vi "GetAcqSeqLeCroy.vi"(0 "Digitizer Settings":T5={"Digitizer delay (us) "=0.0, "rf points per line"=2048, "lines per plane"=128, "Samp Rate (Hz)"=100000000.0, "Additional dig delay (us)"=0.0, "Voltage Scale"=0.4, "Pre-Looks"=0, "Offset delay (us)"=0.0, "bits A/D"=8, "Avg Num"=1, "DigTimeOut"=5.0, "Rel Dig Delay"=0.0, "Dig Ch"=0, "LeCroyCluster"={"LeCroy Channels"=[TRUE, FALSE, FALSE, FALSE], "LC read pt offset"=0.0, "Sweep Avg"=FALSE}, "Main Digitizer"=enum."NI Digitizer", "Dig Config"=enum."Single channel", "Digitizer ID Cluster"={"Acqiris/Alazar/SP ID"=[], "NI Instr Handles"=[], "LeCroy VISA"="", "GaGe Handle"={"Handle"=0, "Sample size"=0, "Resolution"=0, "Offset"=0, "Channels"=0, "Boards"=0}, "ATS Ref"="ATS9350", "Acqiris Address"=["PCI::INSTR0"], "ADQRef"=refnum, "adq_cu_ptr"=refnum}, "Trigger Settings"={"Trig Source"=1, "Trig Coupling"=0, "Trig Slope"=0, "Level (mV)"=1500.0}, "Bulk Acq"=FALSE, "Bulk Start Indexes"=[], "Data Ref RF"=refnum, "NI ID/Channel"=[], "Total Dig CH"=1, "Xtra Ann Trig delay (us)"=10.0, "Fix Z Delay?"=FALSE, "One Way Transmission?"=FALSE, "Data Ref Log"=refnum} {"Trigger Settings"."Trig Slope" items=["Positive", "Negative"]; "Trigger Settings"."Level (mV)" format="%.2f"; "Trigger Settings"."Trig Coupling" items=["DC 1 MOhm", "AC 1 MOhm", "DC 50 Ohm", "AC 50 Ohm"]; "Trigger Settings"."Trig Source" items=["Chan 1", "External"]; "Rel Dig Delay" format="%.2f"; "DigTimeOut" format="%.2f"; "Avg Num" min=1; "Offset delay (us)" format="%.2f"; "Additional dig delay (us)" format="%.2f"; "Digitizer delay (us)" format="%.2f"}, 6 "Motion Settings":T1={"No Motion?"=FALSE, "Motion System"=enum."NI 735x", "Motion Bd ID"=1, "Motion Profile"="SMAC1", "# Axis"=1, "Reverse Z axis?"=TRUE, "SMAC Axis"=0, "scan pair"=enum."y-(x) scan", "RT fps"=6.0, "Steps per mm"=[1000, 1000, 1000, 1000], "Motor Parameters"={"velocity ct/s"=[10000.0, 10000.0, 10000.0, 50000.0], "accel ct/s^2"=[50000.0, 50000.0, 50000.0, 200000.0]}, "One Way Scan"=FALSE, "Reverse One Way Scan"=FALSE, "Global Position (mm)"=[], "Plane"=0, "Distance between\nscan lines (um)"=0.0, "Distance between\nscan planes (um)"=0.0, "number of scan planes"=1, "Total steps in line"=0, "Xtra plane\ndistance  (um)"=100, "Xtra planes "=1, "Add Axis"=FALSE, "overshoot cts"=200, "BKPT Shift"=0, "Scan Start Time (ms)"=0, "ESP VISA"="GPIB::1::INSTR", "3rd Axis"=1, "GL Ref Out"=refnum, "Galil Address"=""} {"3rd Axis" items=["x", "y", "z", "w"]; "Xtra planes" min=1; "Xtra plane\ndistance  (um)" min=0; "Distance between\nscan planes (um)" format="%.2f"; "Distance between\nscan lines (um)" format="%.2f"; "SMAC Axis" items=["None"=0, "Axis 1"=1, "Axis 2"=2, "Axis 3"=3, "Axis 4"=4, "Axis 5"=5, "Axis 6"=6, "Axis 7"=7, "Axis 8"=8, "Vector Space 1"=17, "Vector Space 2"=18, "Vector Space 3"=19, "Vector Space 4"=20]; "Motion Bd ID" min=1 max=32 step=1}, 7 "errorin":errorcluster, 8 "Numbered File":string, 9 "Pop Up":bool, 11 "Source (0: Channel 1)":u16(ring) items=["Channel 1", "Channel 2", "Channel 3", "Channel 4", "Memory 1", "Memory 2", "Memory 3", "Memory 4", "Function 1", "Function 2", "Function 3", "Function 4", "Function 5", "Function 6", "Function 7", "Function 8", "Other"], 14 "save?":bool=TRUE, 15 "Reverse?":bool) -> (17 "Raw VGain (scale)":dbl, 18 "Voltage Scale":T9, 20 "Data Array":i16[][](array[numeric]), 21 "VGain (dB)":dbl, 25 "Ch1 Hz Offset":dbl[](array[numeric]), 26 "Ch2 Hz Offset":dbl[](array[numeric]), 27 "error out":errorcluster)   [LabVIEW 2022 SP3]
uses:
  -DigitizerRoutines/DigitizerSettings.ctl
  -DigitizerRoutines/Digitizer.ctl
  -DigitizerRoutines/DigConfig.ctl
  -DigitizerRoutines/DigitizerID.ctl
  C:/Windows/System32/ADQAPI_dotNet_helper.dll
  Motion Controllers/NI_controller/-NI_MotionRoutines/MotionParameters.ctl
  Motion Controllers/NI_controller/-NI_MotionRoutines/MotionSys.ctl
  Motion Controllers/-MotionRoutines/ScanAxis.ctl
  Motion Controllers/-MotionRoutines/3rdAxis.ctl
  -DigitizerRoutines/DigitizerGlobals.vi
  Motion Controllers/-MotionRoutines/MotionGlobals.vi
  <vilib>/Utility/file.llb/Write Delimited Spreadsheet (DBL).vi
  <instrlib>/LeCroy Wave Series/LeCroy Wave Series.lvlib
panel:
  out "Run Time":sgl
  in  "Timeout (10000 ms)":u32=10000
  in  "Sparsing (0: Every point)":i16
  # "1-D and 2-D B scan settings"
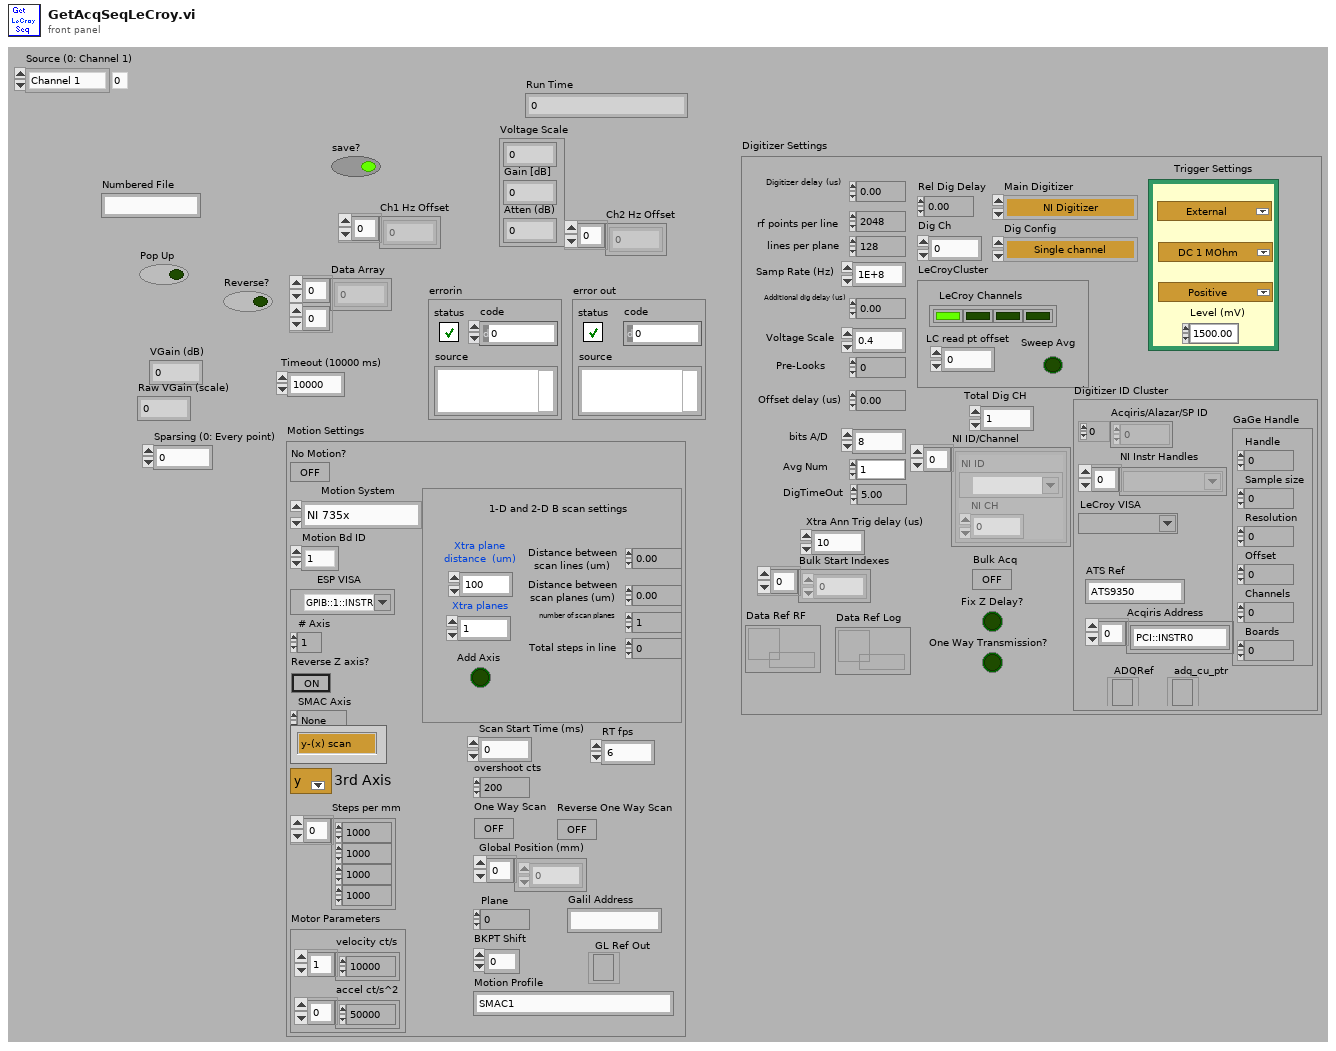
[diagram p1: front panel]
types:
  T1 = typedef "MotionParameters.ctl" = cluster{"No Motion?":bool, "Motion System":T2, "Motion Bd ID":u8, "Motion Profile":string, "# Axis":i8, "Reverse Z axis?":bool, "SMAC Axis":u16, "scan pair":T3, "RT fps":sgl, "Steps per mm":i32[], "Motor Parameters":cluster{"velocity ct/s":dbl[], "accel ct/s^2":dbl[]}, "One Way Scan":bool, "Reverse One Way Scan":bool, "Global Position (mm)":dbl[], "Plane":i32, "Distance between\nscan lines (um)":sgl, "Distance between\nscan planes (um)":sgl, "number of scan planes":i32, "Total steps in line":i32, "Xtra plane\ndistance  (um)":i32, "Xtra planes ":i32, "Add Axis":bool, "overshoot cts":i32, "BKPT Shift":i32, "Scan Start Time (ms)":u32, "ESP VISA":refnum<visa-resource-name>, "3rd Axis":T4, "GL Ref Out":refnum<k7>, "Galil Address":string}
  T2 = typedef "MotionSys.ctl" = enum16{"MM3000", "NI 735x", "Newport ESP", "No Motion Card", "Galil"}
  T3 = typedef "ScanAxis.ctl" = enum16{"y-(x) scan", "x-(y) scan", "z-(x) scan", "z-(y) scan", "y-(z) scan", "x-(z) scan", "w-(x) scan", "w-(y) scan", "w-(z) scan", "x-(w) scan", "y-(w) scan", "z-(w) scan"}
  T4 = typedef "3rdAxis.ctl" = u16
  T5 = typedef "DigitizerSettings.ctl" = cluster{"Digitizer delay (us) ":dbl, "rf points per line":i32, "lines per plane":i32, "Samp Rate (Hz)":dbl, "Additional dig delay (us)":dbl, "Voltage Scale":dbl, "Pre-Looks":i32, "Offset delay (us)":dbl, "bits A/D":i8, "Avg Num":i32, "DigTimeOut":sgl, "Rel Dig Delay":sgl, "Dig Ch":i32, "LeCroyCluster":cluster{"LeCroy Channels":bool[], "LC read pt offset":dbl, "Sweep Avg":bool}, "Main Digitizer":T6, "Dig Config":T7, "Digitizer ID Cluster":T8, "Trigger Settings":cluster{"Trig Source":u16, "Trig Coupling":u16, "Trig Slope":u16, "Level (mV)":dbl}, "Bulk Acq":bool, "Bulk Start Indexes":i32[], "Data Ref RF":refnum<data-value>, "NI ID/Channel":cluster{"NI ID":refnum<k15>, "NI CH":i32}[], "Total Dig CH":i32, "Xtra Ann Trig delay (us)":dbl, "Fix Z Delay?":bool, "One Way Transmission?":bool, "Data Ref Log":refnum<data-value>}
  T6 = typedef "Digitizer.ctl" = enum16{"Acqiris Digitizer", "NI Digitizer", "LeCroy", "GaGe", "AlazarTech", "No Digitizer", "Teledyne"}
  T7 = typedef "DigConfig.ctl" = enum16{"Single channel", "2 Chans w/ 2 Acqiris", "2 Chans w/ 1 Acqiris", "5-CH Pulser New", "5-CH pulser w/ ann array", "5-pass style ann array", "Empty"}
  T8 = typedef "DigitizerID.ctl" = cluster{"Acqiris/Alazar/SP ID":u32[], "NI Instr Handles":refnum<k15>[], "LeCroy VISA":refnum<visa-resource-name>, "GaGe Handle":cluster{"Handle":u32, "Sample size":u32, "Resolution":i32, "Offset":i32, "Channels":u32, "Boards":u32}, "ATS Ref":string, "Acqiris Address":string[], "ADQRef":refnum<k24>, "adq_cu_ptr":refnum<k24>}
  T9 = cluster{sgl, "Gain [dB]  ":sgl, "Atten (dB)":sgl}
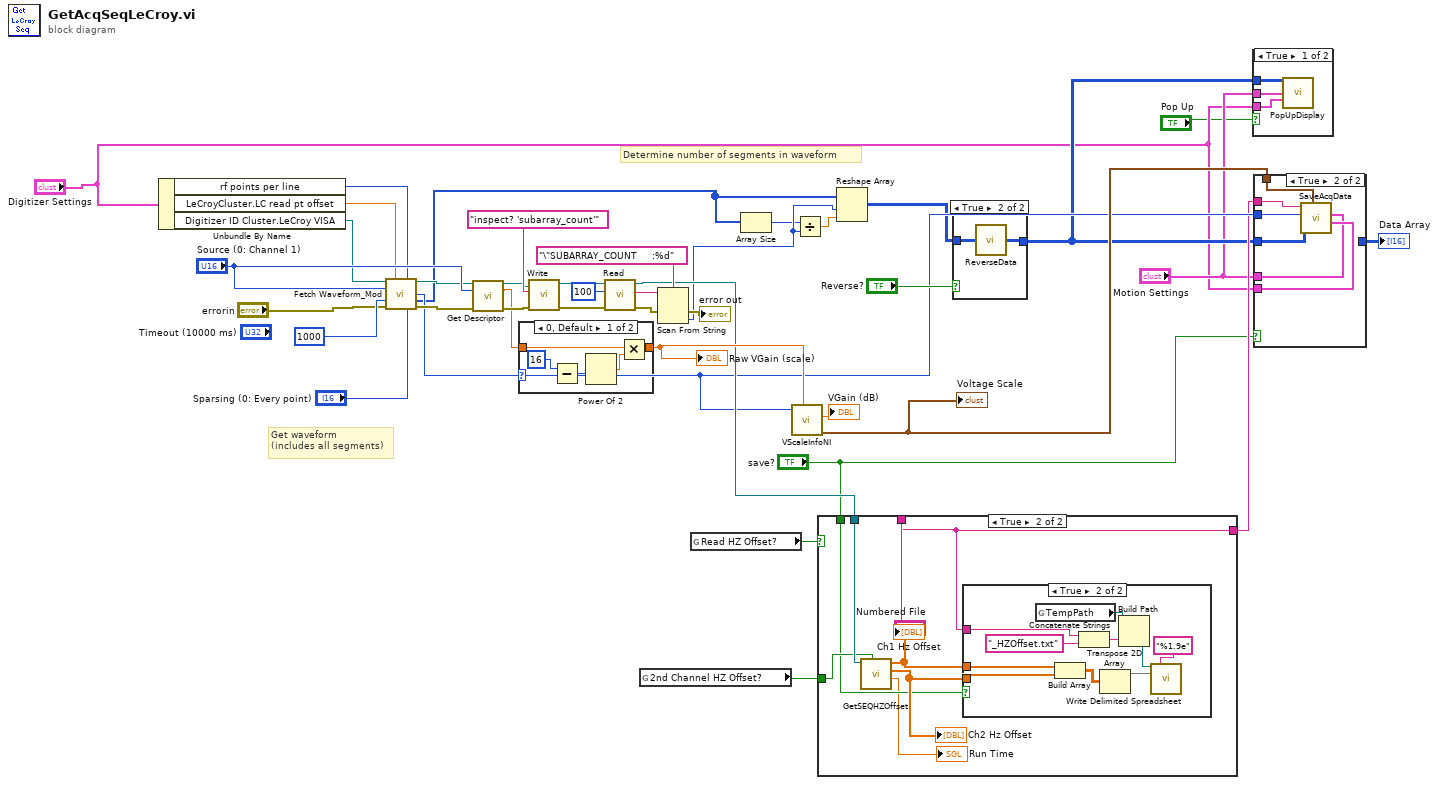
[diagram p0: block diagram]
diagram:
  # "Determine number of segments in waveform"
  # "Get waveform\n(includes all segments)"
  n1 = Unbundle By Name("Digitizer Settings") -> ("rf points per line"=w20:i32, "LeCroyCluster.LC read pt offset"=w19:dbl, "Digitizer ID Cluster.LeCroy VISA"=w18:refnum<visa-resource-name>)
  n2 = call "Fetch Waveform_Mod.vi"("VISA resource name"=w18, "First point (0: First point)"=w19, "Number of points (0: All points)"=w20, "Source (0: Channel 1)"="Source (0: Channel 1)", "Timeout (10000 ms)"=u32 1000, "error in (no error)"="errorin", "Sparsing (0: Every point)"="Sparsing (0: Every point)") -> ("VISA resource name out"=w17:refnum<visa-resource-name>, "Nom_Bits"=w12:i16, "Raw Data"=w8:i16[], "error out"=w24:errorcluster)  [unwired: 3 in, 2 out]
  n3 = call <instrlib>:"Get Descriptor.vi"("VISA resource name"=w17, "Source (0: Channel 1)"="Source (0: Channel 1)", "error in (no error)"=w24) -> ("VISA resource name out"=w29:refnum<visa-resource-name>, "Vertical gain"=w22:sgl, "error out"=w28:errorcluster)  [unwired: 2 in, 8 out]
  n4 = case shown="0, Default" w12 {
    selector: w12 -> [w45 _]
    tunnel: w22 -> [w46 w48]
    tunnel: [w47 w48] -> w21
    frame 0, Default {
      n5 = Subtract(x=16, y=w45) -> (x-y=w43:i32)
      n6 = Power Of 2(x=w43) -> (2^x=w42:dbl)
      n7 = Multiply(x=w46, y=w42) -> (x*y=w47:dbl)
    }
    frame 8 {
    }
  }
  "Raw VGain (scale)" <- w21
  n8 = call <instrlib>:"Write.vi"("error in (no error)"=w28, "Write Buffer"="inspect? 'subarray_count'", "VISA resource name"=w29) -> ("error out"=w37:errorcluster, "VISA resource name out"=w35:refnum<visa-resource-name>)  [unwired: 6 in, 1 out]
  n9 = call <instrlib>:"Read.vi"("error in (no error)"=w37, "Byte Count"=u32 100, "VISA resource name"=w35) -> ("error out"=w41:errorcluster, "Read Buffer"=w39:string, "VISA resource name out"=w16:refnum<visa-resource-name>)  [unwired: 5 in, 1 out]
  n10 = global read "DigitizerGlobals.vi" "2nd Channel HZ Offset?"() -> (w14:bool)
  n11 = Scan From String(format string="\"SUBARRAY_COUNT     :%d", input string=w39, error in=w41) -> (error out=→"error out":errorcluster, output 1=w9:i32)  [unwired: 2 in, 2 out]
  n12 = global read "DigitizerGlobals.vi" "Read HZ Offset?"() -> (w15:bool)
  n13 = Array Size(array=w8) -> (size(s)=w2:i32)
  n14 = call "VScaleInfoNI.vi"("A/D bits"=w12, "gain"=w21) -> ("vGain (dB)"=→"VGain (dB)":dbl, "Voltage Scale"=w31:T9)  [unwired: 5 in, 2 out]
  "Voltage Scale" <- w31
  n15 = Divide(x=w2, y=w9) -> (x/y=w1:dbl)
  n16 = case shown="True" w15 {
    tunnel: w16 -> [_ w56]
    tunnel: w14 -> [_ w55]
    tunnel: "save?" -> [_ w52]
    tunnel: "Numbered File" -> [w49 w50]
    tunnel: [w49 w50] -> w11
    frame False {
    }
    frame True {
      n17 = call "GetSEQHZOffset.vi"("2nd Channel?"=w55, "VISA resource name"=w56) -> ("Run Time (s)"=→"Run Time":sgl, "CH2 HZ OFFSET"=w53:dbl[], "CH1 HZ OFFSET"=w54:dbl[])  [unwired: 4 in, 1 out]
      "Ch1 Hz Offset" <- w54
      "Ch2 Hz Offset" <- w53
      n18 = case shown="True" w52 {
        tunnel: w54 -> [_ w61]
        tunnel: w53 -> [_ w59]
        tunnel: w50 -> [_ w66]
        frame False {
        }
        frame True {
          n19 = global read "MotionGlobals.vi" "TempPath"() -> (w63:path)
          n20 = Build Array(w61, w59) -> (w60:dbl[][])
          n21 = Concatenate Strings(w66, "_HZOffset.txt" ("string")) -> (w64:string)
          n22 = Transpose 2D Array(2D array=w60) -> (transposed array=w57:dbl[][])
          n23 = Build Path(base path=w63, name or relative path=w64) -> (appended path=w62:path)
          n24 = call-poly <vilib>:"Write Delimited Spreadsheet.vi"("file path (dialog if empty)"=w62, "format (%.3f)"="%1.9e", "2D data"=w57) -> ()  [unwired: 11 in, 2 out]
        }
      }
    }
  }
  n25 = Reshape Array(w8, w9, w1) -> (w7:i16[][])
  n26 = case shown="True" "Reverse?" {
    tunnel: w7 -> [w67 w69]
    tunnel: [w67 w68] -> w6
    frame False {
    }
    frame True {
      n27 = call "ReverseData.vi"("Array in"=w69) -> ("Array out"=w68:i16[][])
    }
  }
  n28 = case shown="True" "Pop Up" {
    tunnel: w6 -> [w72 _]
    tunnel: "Motion Settings" -> [w71 _]
    tunnel: "Digitizer Settings" -> [w70 _]
    frame True {
      n29 = call "PopUpDisplay.vi"("Data"=w72, "Motion Settings In"=w71, "Digitizer Settings"=w70) -> ()  [unwired: 13 in]
    }
    frame False {
    }
  }
  n30 = case shown="True" "save?" {
    tunnel: w12 -> [_ w79]
    tunnel: w6 -> [w73 w78]
    tunnel: [w73 _] -> w26
    tunnel: w11 -> [_ w77]
    tunnel: w31 -> [_ w76]
    tunnel: "Digitizer Settings" -> [_ w75]
    tunnel: "Motion Settings" -> [_ w74]
    frame False {
    }
    frame True {
      n31 = call "SaveAcqData.vi"("Digitizer Settings"=w75, "Motion Settings"=w74, "Votage scaling"=w76, "Array"=w78, "Dig Word Size"=w79, "File Name"=w77) -> ()  [unwired: 5 in]
    }
  }
  "Data Array" <- w26
